vi "Window-controller response_v1.vi"() -> ()   [LabVIEW 2020]
panel:
  out "OutPut  (Free Index)":T1(array[cluster]) {"Return Command" items=["load_plane_complete_c"=32, "load_points_complete_c"=38, "run_plane_complete_c"=45, "run_points_complete_c"=39, "run_frequency_complete_c"=40, "Stim_time"=47, "Unrecognised"=0]}
  out "OutPut":T1(array[cluster]) {"Return Command" items=["load_plane_complete_c"=32, "load_points_complete_c"=38, "run_plane_complete_c"=45, "run_points_complete_c"=39, "run_frequency_complete_c"=40, "Stim_time"=47, "Unrecognised"=0]}
  out "timed out?":bool
  in  "error in (no error) 2":errorcluster
  out "Numeric":i32
  out "after substring":string
  out "offset past match":i32
  out "match substring":string
  out "before substring":string
  in  "error in (no error)":errorcluster
  in  "stop":bool
  out "Timeout":bool
  # "(Index locked, latest 5 messages)"
  # "Winpcap"
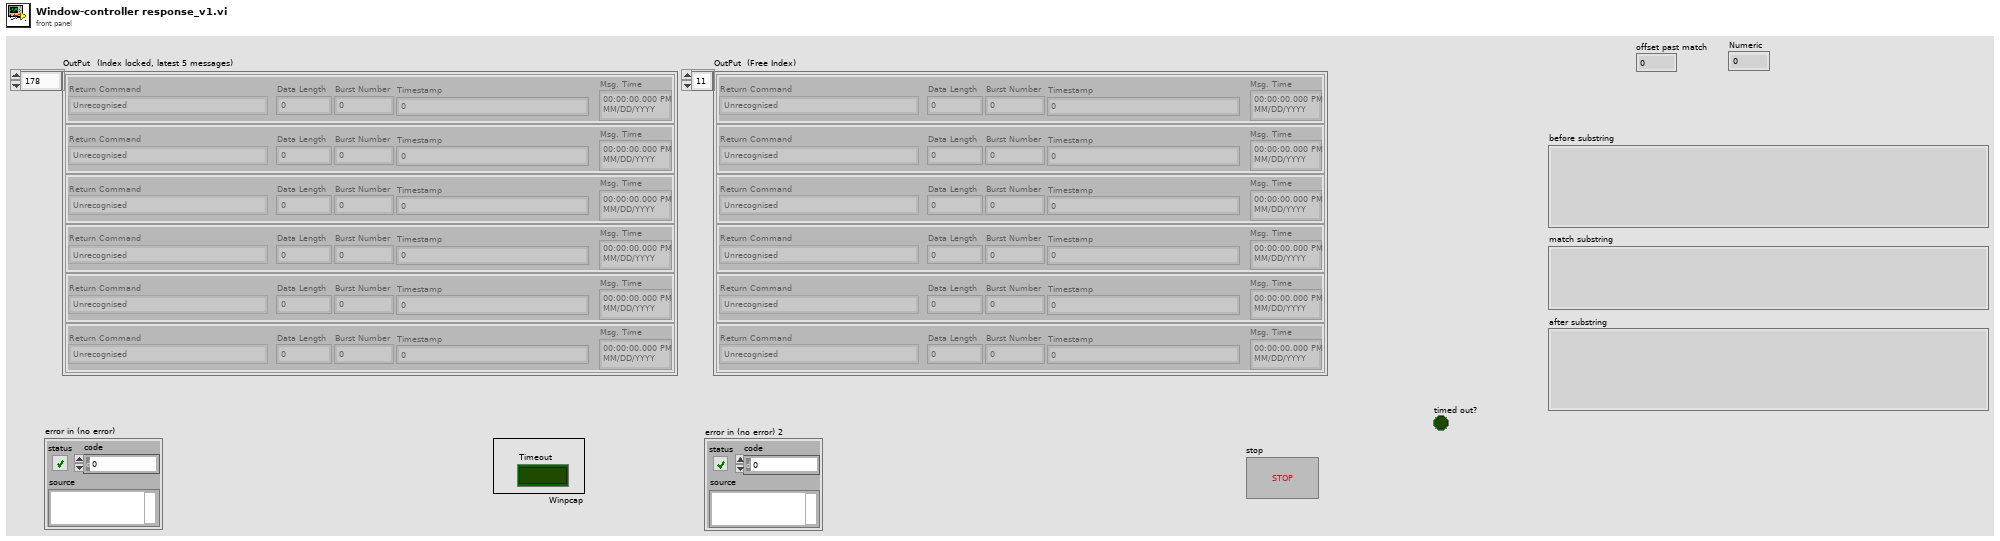
[diagram p1: front panel]
types:
  T1 = cluster{"Return Command":u16, "Data Length":u32, "Burst Number":u32, "Timestamp":u32, "Msg. Time":timestamp}[]
  T2 = cluster{"String":string, "Time stamp":timestamp}[]
  T3 = cluster{"Return Command":u16, "Data Length":u32, "Burst Number":u32, "Timestamp":u32, "Msg. Time":timestamp}
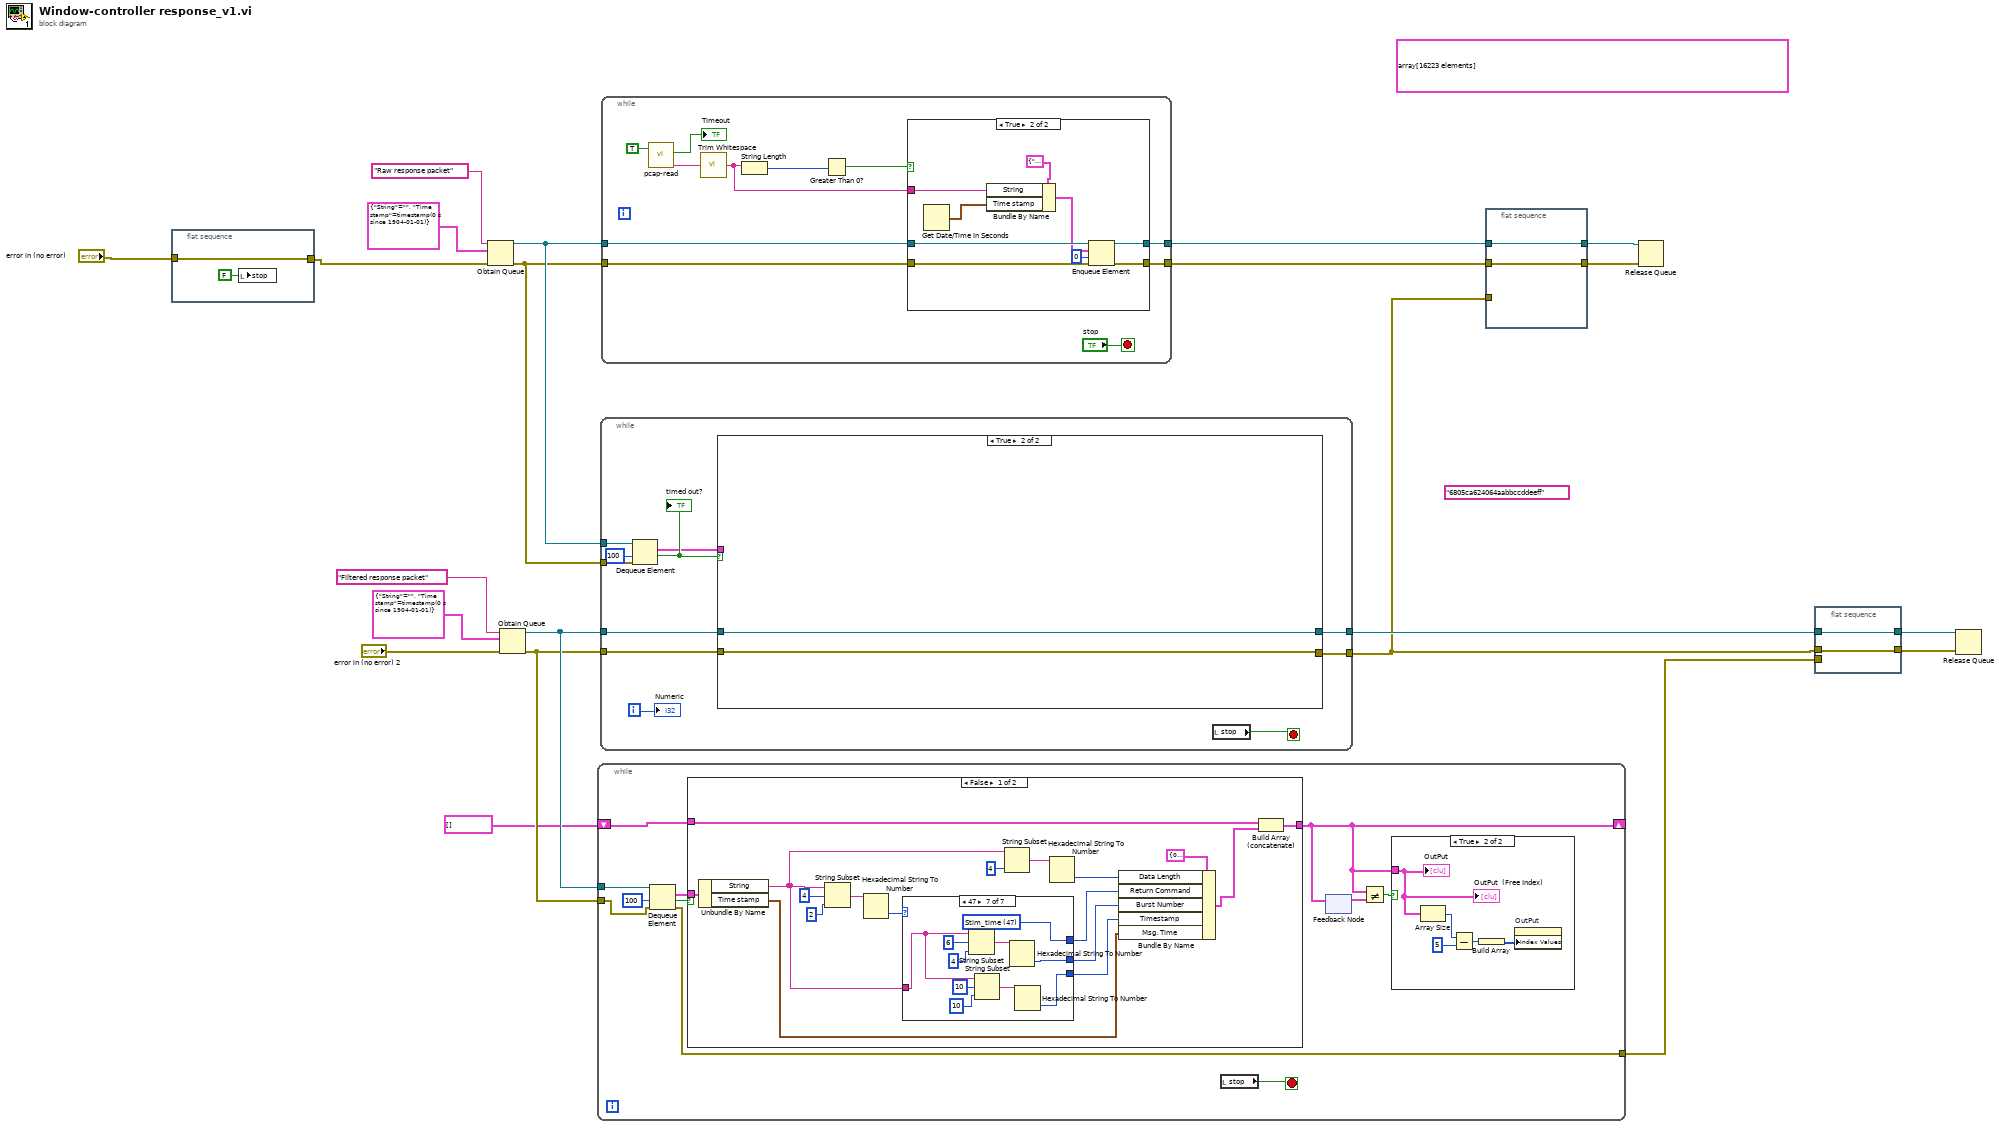
[diagram p0: block diagram]
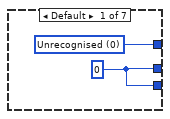
[diagram p3: hidden frame]
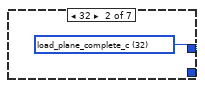
[diagram p4: hidden frame]
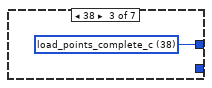
[diagram p5: hidden frame]
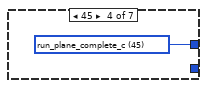
[diagram p6: hidden frame]
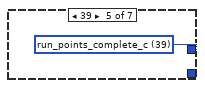
[diagram p7: hidden frame]
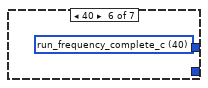
[diagram p8: hidden frame]
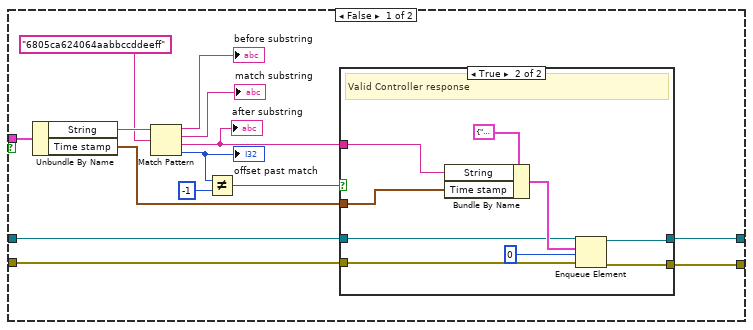
[diagram p10: hidden frame]
diagram:
  (unwired) "6805ca624064aabbccddeeff"
  (unwired) T2 array[16223 elements]
  n1 = flat-sequence {
    tunnel: "error in (no error)" -> [w22]
    tunnel: [w22] -> w1
    frame #0 {
      n2 = local write "stop"(FALSE ("stop")) -> ()
    }
  }
  n3 = Obtain Queue(name (unnamed)="Raw response packet", element data type=cluster{"String":string, "Time stamp":timestamp} {"String"="", "Time stamp"=timestamp(0 s since 1904-01-01)}, error in (no error)=w1) -> (queue out=w19:refnum<queue>, error out=w18:errorcluster)  [unwired: 2 in, 1 out]
  n4 = Obtain Queue(name (unnamed)="Filtered response packet", element data type=cluster{"String":string, "Time stamp":timestamp} {"String"="", "Time stamp"=timestamp(0 s since 1904-01-01)}, error in (no error)="error in (no error) 2") -> (queue out=w14:refnum<queue>, error out=w13:errorcluster)  [unwired: 2 in, 1 out]
  n5 = while {
    tunnel: w14 -> [w33]
    tunnel: w13 -> [w32]
    shift-right: [w25] -> _
    shift-left: T1 [] -> [w28]
    tunnel: [w24] -> w3
    stop <- w29 stop-if-true
    n6 = Dequeue Element(queue=w33, timeout in ms (-1)=100, error in (no error)=w32) -> (element=w30:cluster{"String":string, "Time stamp":timestamp}, timed out?=w31:bool, error out=w24:errorcluster)  [unwired: 1 out]
    n7 = case shown="False" w31 {
      tunnel: w30 -> [w46 _]
      tunnel: w28 -> [w43 w74]
      tunnel: [w41 w74] -> w25
      frame False {
        n8 = Unbundle By Name(w46) -> ("String"=w44:string, "Time stamp"=w40:timestamp)
        n9 = String Subset(string=w44, offset (0)=4, length (rest)=2 ("length (rest)")) -> (substring=w54:string)
        n10 = Hexadecimal String To Number(string=w54) -> (number=w52:u32)  [unwired: 2 in, 1 out]
        n11 = case shown="47" w52 {
          tunnel: [w58 w59 w60 w61 w62 w63 w73] -> w49
          tunnel: w44 -> [_ _ _ _ _ _ w66]
          tunnel: [w57 _ _ _ _ _ w69] -> w48
          tunnel: [w57 _ _ _ _ _ w64] -> w47
          frame Default {
            w57 = u32 0
            w58 = u16 0 items=["load_plane_complete_c"=32, "load_points_complete_c"=38, "run_plane_complete_c"=45, "run_points_complete_c"=39, "run_frequency_complete_c"=40, "Stim_time"=47, "Unrecognised"=0]
          }
          frame 32 {
            w59 = u16 32 items=["load_plane_complete_c"=32, "load_points_complete_c"=38, "run_plane_complete_c"=45, "run_points_complete_c"=39, "run_frequency_complete_c"=40, "Stim_time"=47, "Unrecognised"=0]
          }
          frame 38 {
            w60 = u16 38 items=["load_plane_complete_c"=32, "load_points_complete_c"=38, "run_plane_complete_c"=45, "run_points_complete_c"=39, "run_frequency_complete_c"=40, "Stim_time"=47, "Unrecognised"=0]
          }
          frame 45 {
            w61 = u16 45 items=["load_plane_complete_c"=32, "load_points_complete_c"=38, "run_plane_complete_c"=45, "run_points_complete_c"=39, "run_frequency_complete_c"=40, "Stim_time"=47, "Unrecognised"=0]
          }
          frame 39 {
            w62 = u16 39 items=["load_plane_complete_c"=32, "load_points_complete_c"=38, "run_plane_complete_c"=45, "run_points_complete_c"=39, "run_frequency_complete_c"=40, "Stim_time"=47, "Unrecognised"=0]
          }
          frame 40 {
            w63 = u16 40 items=["load_plane_complete_c"=32, "load_points_complete_c"=38, "run_plane_complete_c"=45, "run_points_complete_c"=39, "run_frequency_complete_c"=40, "Stim_time"=47, "Unrecognised"=0]
          }
          frame 47 {
            w73 = u16 47 items=["load_plane_complete_c"=32, "load_points_complete_c"=38, "run_plane_complete_c"=45, "run_points_complete_c"=39, "run_frequency_complete_c"=40, "Stim_time"=47, "Unrecognised"=0]
            n12 = String Subset(string=w66, offset (0)=6, length (rest)=4 ("length (rest)")) -> (substring=w70:string)
            n13 = String Subset(string=w66, offset (0)=10, length (rest)=10 ("length (rest)")) -> (substring=w68:string)
            n14 = Hexadecimal String To Number(string=w70) -> (number=w69:u32)  [unwired: 2 in, 1 out]
            n15 = Hexadecimal String To Number(string=w68) -> (number=w64:u32)  [unwired: 2 in, 1 out]
          }
        }
        n16 = String Subset(string=w44, length (rest)=4 ("length (rest)")) -> (substring=w55:string)  [unwired: 1 in]
        n17 = Hexadecimal String To Number(string=w55) -> (number=w50:u32)  [unwired: 2 in, 1 out]
        n18 = Bundle By Name(cluster=T3 {"Return Command"=0, "Data Length"=0, "Burst Number"=0, "Timestamp"=0, "Msg. Time"=timestamp(0 s since 1904-01-01)} ("Cluster 2"), "Data Length"=w50, "Return Command"=w49, "Burst Number"=w48, "Timestamp"=w47, "Msg. Time"=w40) -> (w42:T3)
        n19 = Build Array (concatenate)(w43, w42) -> (w41:T1)
      }
      frame True {
      }
    }
    n20 = local read "stop"() -> (w29:bool)
    n21 = feedback-in #1(w25) -> ()
    n22 = feedback #1() -> (w26:T1)  [unwired: 1 in]
    n23 = Not Equal?(x=w25, y=w26) -> (x != y?=w27:bool)
    n24 = case shown="True" w27 {
      tunnel: w25 -> [_ w35]
      frame False {
      }
      frame True {
        n25 = Array Size(array=w35) -> (size(s)=w39:i32)
        n26 = Subtract(x=w39, y=5) -> (x-y=w37:i32)
        n27 = Build Array(w37) -> (w36:i32[])
        n28 = property on="OutPut" class="Arr (strict)"("Index Values"=w36) -> ()  [unwired: 2 in, 2 out]
        "OutPut" <- w35
        "OutPut  (Free Index)" <- w35
      }
    }
  }
  n29 = while {
    tunnel: w19 -> [w85]
    tunnel: w18 -> [w84]
    tunnel: w13 -> [w78]
    tunnel: w14 -> [w77]
    tunnel: [w76] -> w6
    tunnel: [w75] -> w7
    i -> [w79]
    stop <- w80 stop-if-true
    n30 = Dequeue Element(queue=w85, timeout in ms (-1)=100, error in (no error)=w84) -> (element=w81:cluster{"String":string, "Time stamp":timestamp}, timed out?=w82:bool)  [unwired: 2 out]
    "timed out?" <- w82
    n31 = case shown="True" w82 {
      tunnel: w81 -> [w99 _]
      tunnel: w78 -> [w91 w112]
      tunnel: w77 -> [w90 w111]
      tunnel: [w87 w112] -> w76
      tunnel: [w86 w111] -> w75
      frame False {
        n32 = Unbundle By Name(w99) -> ("String"=w96:string, "Time stamp"=w88:timestamp)
        n33 = Match Pattern(string=w96, regular expression="6805ca624064aabbccddeeff" ("string")) -> (before substring=→"before substring":string, match substring=→"match substring":string, after substring=w89:string, offset past match=w94:i32)  [unwired: 1 in]
        "offset past match" <- w94
        "after substring" <- w89
        n34 = Not Equal?(x=w94, y=-1) -> (x != y?=w92:bool)
        n35 = case shown="True" w92 {
          tunnel: w91 -> [w101 w104]
          tunnel: w90 -> [w100 w105]
          tunnel: w89 -> [_ w107]
          tunnel: w88 -> [_ w106]
          tunnel: [w101 w103] -> w87
          tunnel: [w100 w102] -> w86
          frame False {
            # "Not a controller response"
          }
          frame True {
            # "Valid Controller response"
            n36 = Bundle By Name(cluster=cluster{"String":string, "Time stamp":timestamp} {"String"="", "Time stamp"=timestamp(0 s since 1904-01-01)}, "String"=w107, "Time stamp"=w106) -> (w109:cluster{"String":string, "Time stamp":timestamp})
            n37 = Enqueue Element(queue=w105, element=w109, timeout in ms (-1)=0, error in (no error)=w104) -> (queue out=w102:refnum<queue>, error out=w103:errorcluster)  [unwired: 1 out]
          }
        }
      }
      frame True {
      }
    }
    n38 = local read "stop"() -> (w80:bool)
    "Numeric" <- w79
  }
  n39 = while {
    tunnel: w18 -> [w119]
    tunnel: w19 -> [w120]
    tunnel: [w118] -> w11
    tunnel: [w117] -> w10
    stop <- "stop" stop-if-true
    n40 = call "pcap-read.vi"("Opened"=TRUE) -> ("Timeout"=→"Timeout":bool, "Packet Data:"=w114:string)  [unwired: 5 out]
    n41 = call <vilib>:"Trim Whitespace.vi"("string"=w114) -> ("trimmed string"=w121:string)  [unwired: 1 in]
    n42 = String Length(string=w121) -> (length=w113:i32)
    n43 = Greater Than 0?(x=w113) -> (x > 0?=w122:bool)
    n44 = case shown="True" w122 {
      tunnel: w121 -> [_ w134]
      tunnel: w120 -> [w125 w130]
      tunnel: w119 -> [w124 w131]
      tunnel: [w124 w128] -> w118
      tunnel: [w125 w127] -> w117
      frame False {
      }
      frame True {
        n45 = Get Date/Time In Seconds() -> (seconds since 1Jan1904=w132:timestamp)
        n46 = Bundle By Name(cluster=cluster{"String":string, "Time stamp":timestamp} {"String"="", "Time stamp"=timestamp(0 s since 1904-01-01)}, "String"=w134, "Time stamp"=w132) -> (w129:cluster{"String":string, "Time stamp":timestamp})
        n47 = Enqueue Element(queue=w130, element=w129, timeout in ms (-1)=0, error in (no error)=w131) -> (queue out=w127:refnum<queue>, error out=w128:errorcluster)  [unwired: 1 out]
      }
    }
  }
  n48 = flat-sequence {
    tunnel: w11 -> [w135]
    tunnel: w10 -> [w136]
    tunnel: [w136] -> w9
    tunnel: [w135] -> w8
    tunnel: w6 -> [_]
    frame #0 {
    }
  }
  n49 = Release Queue(queue=w9, error in (no error)=w8) -> ()  [unwired: 1 in, 3 out]
  n50 = flat-sequence {
    tunnel: w7 -> [w138]
    tunnel: w6 -> [w137]
    tunnel: [w138] -> w5
    tunnel: [w137] -> w4
    tunnel: w3 -> [_]
    frame #0 {
    }
  }
  n51 = Release Queue(queue=w5, error in (no error)=w4) -> ()  [unwired: 1 in, 3 out]
